vi "Send Enqueuer to Core.vi"(8 "error in (no error)":errorcluster, 10 "Client/Service Enqueuer":refnum<class "Message Enqueuer.lvclass">, 11 "WS Test Client in":refnum<class "WS Test Client.lvclass">) -> (0 "error out":errorcluster, 3 "WS Test Client out":refnum<class "WS Test Client.lvclass">)   [LabVIEW 2016, in "Echo Broadcast Test Without Server Manager.lvlib" / "WS Test Client.lvclass"]
uses:
  WS Test Client.lvclass
  <vilib>/ActorFramework/Message Enqueuer/Message Enqueuer.lvclass
  WS Test Client.lvclass/WS Test Client.ctl
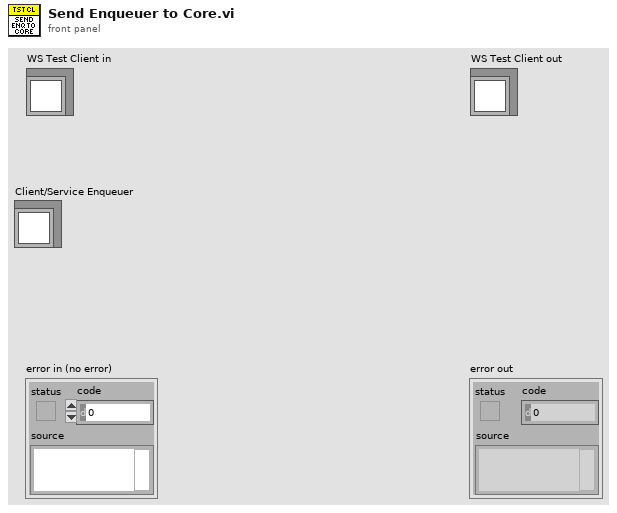
[diagram p1: front panel]
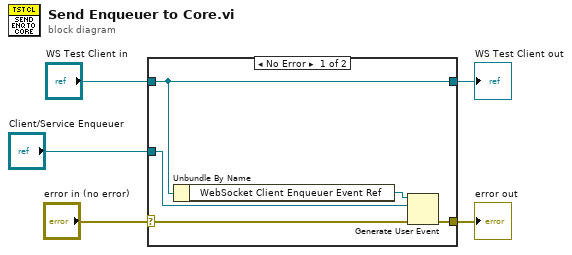
[diagram p0: block diagram]
diagram:
  n1 = case shown="No Error" "error in (no error)" {
    selector: "error in (no error)" -> [w7 w12]
    tunnel: [w6 w12] -> w4
    tunnel: [w10 w11] -> w2
    tunnel: "WS Test Client in" -> [w10 w11]
    tunnel: "Client/Service Enqueuer" -> [w8 _]
    frame No Error {
      n2 = Unbundle By Name(w10) -> ("WebSocket Client Enqueuer Event Ref"=w9:refnum<user-event>)
      n3 = Generate User Event(user event=w9, event data cluster=w8, error in=w7) -> (error out=w6:errorcluster)  [unwired: 1 in, 1 out]
    }
    frame Error {
    }
  }
  "error out" <- w4
  "WS Test Client out" <- w2
